vi "LV3Climb.vi"(7 "Deactivate?":bool, 8 "error in (no error)":errorcluster, 9 "Activate?":bool, 10 "Reclimb?":bool, 11 "Elevator Concrete in":refnum<class "Elevator Concrete.lvclass">) -> (0 "error out":errorcluster, 1 "activate wrist lock":bool, 3 "Elevator Concrete out":refnum<class "Elevator Concrete.lvclass">)   [LabVIEW 2018, in "Elevator.lvlib" / "Elevator Concrete.lvclass"]
uses:
  Elevator Concrete.lvclass
  C:/Users/Public/Documents/2019DeepSpace/Classes/Elevator/Elevator.lvclass
  Elevator States Climb.ctl
  Elevator.lvclass/Elevator.ctl
  <vilib>/Rock Robotics/WPI/ThirdParty/Phoenix-LabVIEW/Motor Controller/Controls/CTRE_Phoenix_MotorControl_ControlMode.ctl
  Elevator Concrete.lvclass/Elevator Concrete.ctl
  Public Methods/Read Arm Position Values.vi
  <vilib>/Rock Robotics/WPI/ThirdParty/Phoenix-LabVIEW/Motor Controller/Get/CTRE_Phoenix_MotorController_GetQuadratureData.vi
  <vilib>/Rock Robotics/Network Tables/NT Write String.vi
  Elevator.lvclass
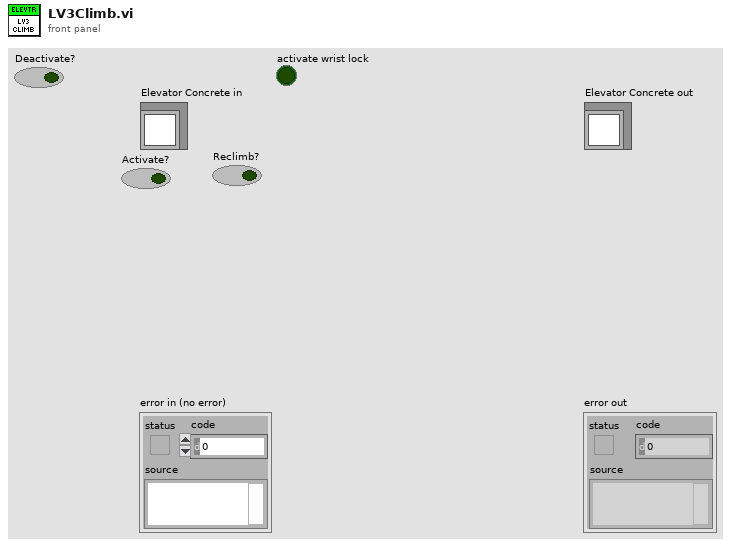
[diagram p1: front panel]
types:
  T1 = typedef "Elevator.lvlib/Elevator.lvclass/Elevator States Climb.ctl" = enum16{"Pre-Lift", "Deploy", "Activate Suction", "Climb", "Climbed", "Unclimb", ""}
  T2 = typedef "Elevator.lvlib/Elevator.lvclass/Elevator Constants.ctl" = cluster{"Arm Motion Magic Max Velocity":u32, "Arm Motion Magic Max Acceleration":u32, "Wrist Motion Magic Max Velocity":u32, "Wrist Motion Magic Max Acceleration":u32, "Arm Gear Ratio":dbl, "Wrist Gear Ratio":dbl, "Arm Encoder ABS Value":i32, "Wrist Encoder ABS Value":i32}
  T3 = typedef "Elevator.lvlib/Elevator.lvclass/Arm Position Values.ctl" = cluster{"C0 Arm":dbl, "C1 Arm":dbl, "C2 Arm":dbl, "H1 Arm":dbl, "H2 Arm":dbl, "C0 Wrist":dbl, "C1 Wrist ":dbl, "C2 Wrist":dbl, "H1 Wrist":dbl, "H2 Wrist":dbl, "Deploy Arm":dbl, "Deploy Wrist":dbl, "Climb Arm":dbl, "Climb Wrist":dbl, "Stowed Arm":dbl, "Stowed Wrist":dbl}
  T4 = typedef "CTRE_Phoenix_MotorControl_ControlMode.ctl" = u16
  T5 = typedef "WPI_MotorControlDeviceRef.ctl" = cluster{"DeviceStatus":errorcluster, "Type":T6, "PWM":cluster{"PWM Channel":T7, "DeadBand":T8}, "CAN":cluster{"Device Number":u8, "SetOutput VI Ref":variant, "GetOutput VI Ref":variant, "Enable VI Ref":variant, "Disable VI Ref":variant, "Data":variant}, "Invert":bool, "DIO PWM":cluster{"PWM \"Enable\" Channel":T7, "DIOChannel":T9, "PWM Rate":dbl}}
  T6 = typedef "WPI_MotorControlType.ctl" = enum16{"PWM", "CAN", "DIO PWM"}
  T7 = typedef "FPGA_DIOPWMChannel.ctl" = enum8{"PWM 0", "PWM 1", "PWM 2", "PWM 3", "PWM 4", "PWM 5", "PWM 6", "PWM 7", "PWM 8", "PWM 9", "PWM MXP 0", "PWM MXP 1", "PWM MXP 2", "PWM MXP 3", "PWM MXP 4", "PWM MXP 5", "PWM MXP 6", "PWM MXP 7", "PWM MXP 8", "PWM MXP 9", "Invalid"}
  T8 = typedef "WPI_PWMDeadband.ctl" = cluster{"Name":string, "maxPositivePwm":i32, "minPositivePwm":i32, "centerPwm":i32, "maxNegativePwm":i32, "minNegativePwm":i32, "angularRange":u16}
  T9 = typedef "FPGA_DIOChannel.ctl" = enum8{"DIO 0", "DIO 1", "DIO 2", "DIO 3", "DIO 4", "DIO 5", "DIO 6", "DIO 7", "DIO 8", "DIO 9", "DIO MXP 0", "DIO MXP 1", "DIO MXP 2", "DIO MXP 3", "DIO MXP 4", "DIO MXP 5", "DIO MXP 6", "DIO MXP 7", "DIO MXP 8", "DIO MXP 9", "DIO MXP 10", "DIO MXP 11", "DIO MXP 12", "DIO MXP 13", "DIO MXP 14", "DIO MXP 15", "SPI Port CS1", "SPI Port CS2", "SPI Port CS3", "SPI Port MISO", "SPI Port MOSI", "Invalid"}
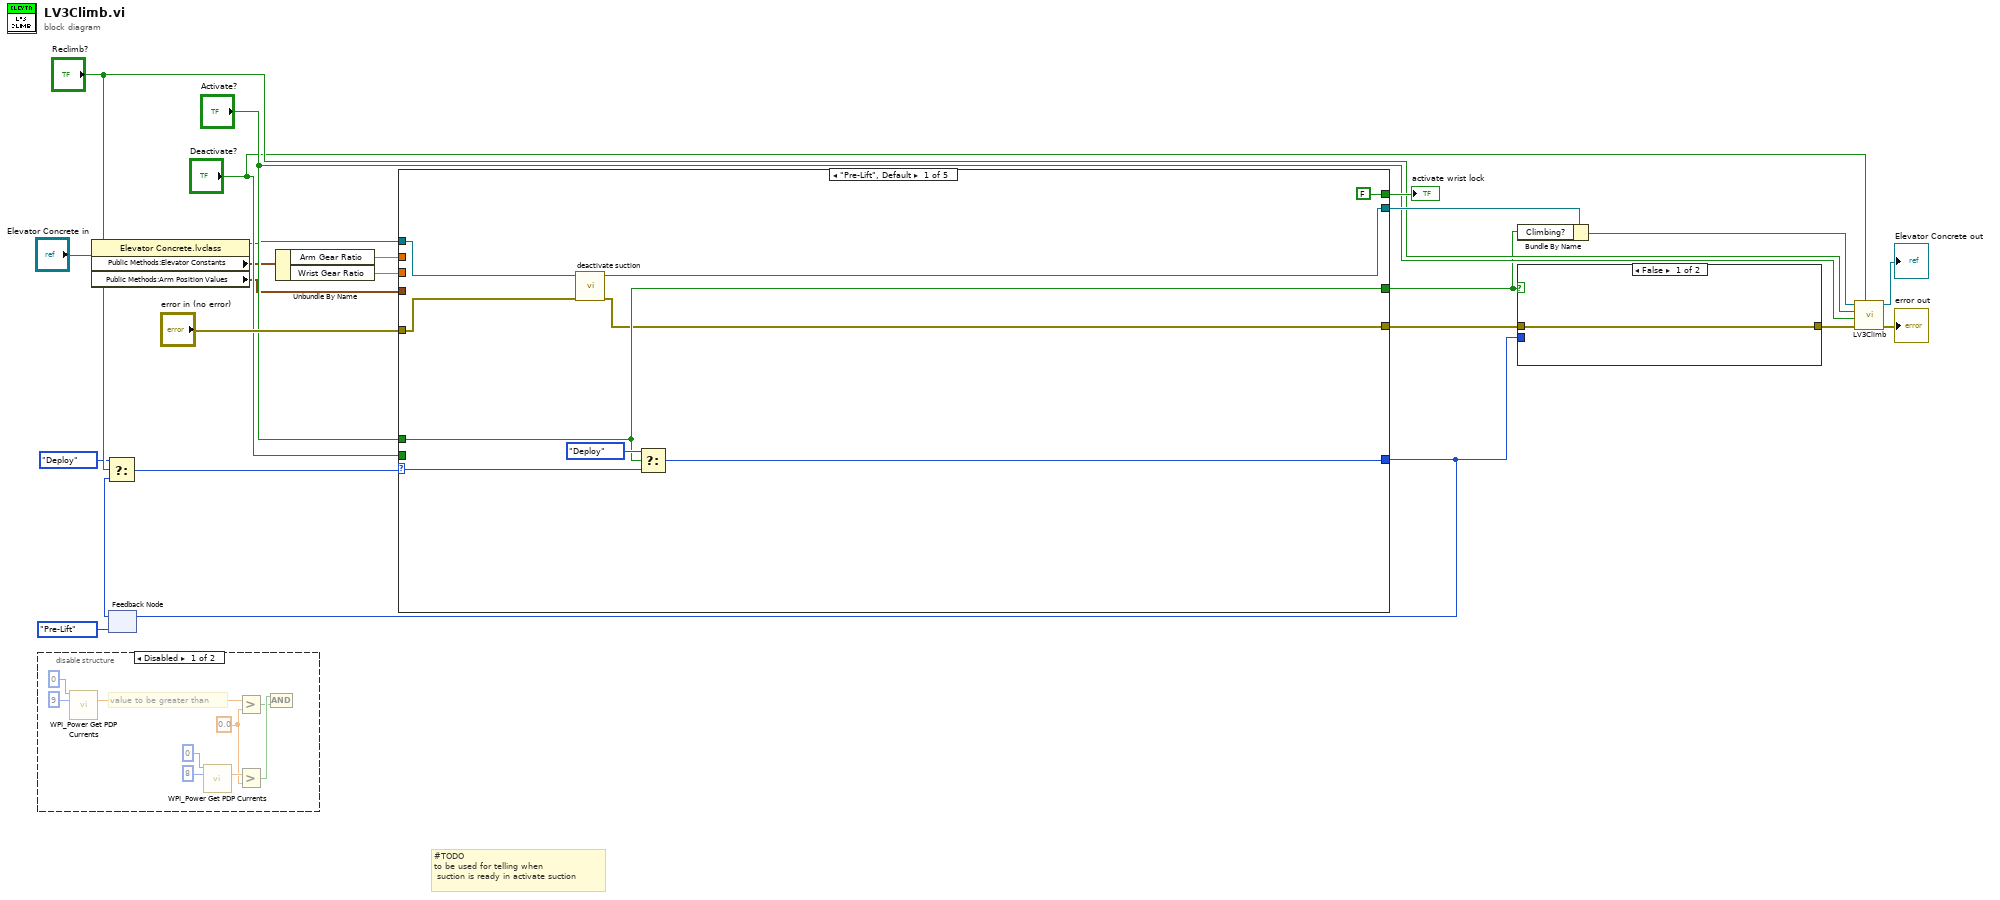
[diagram p0: block diagram]
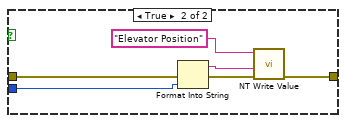
[diagram p2: hidden frame]
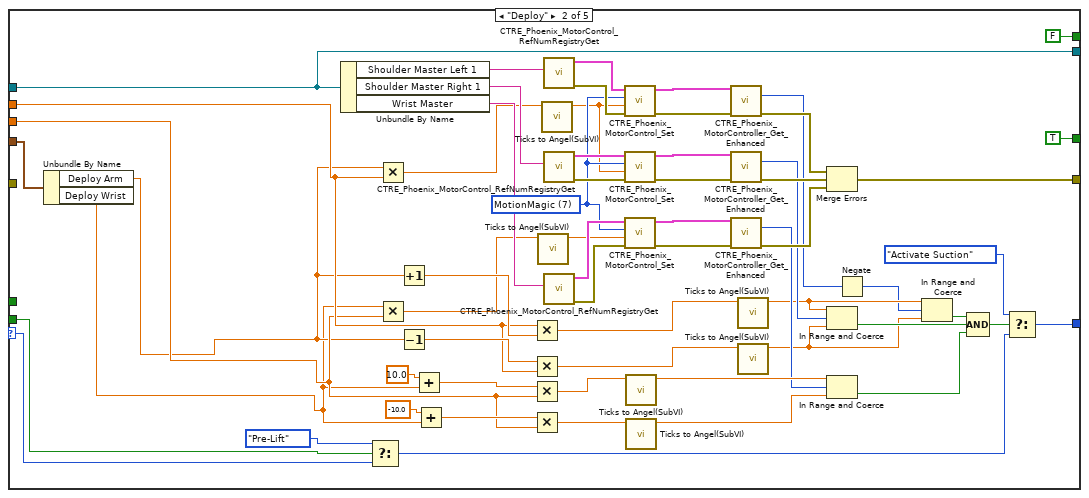
[diagram p4: hidden frame]
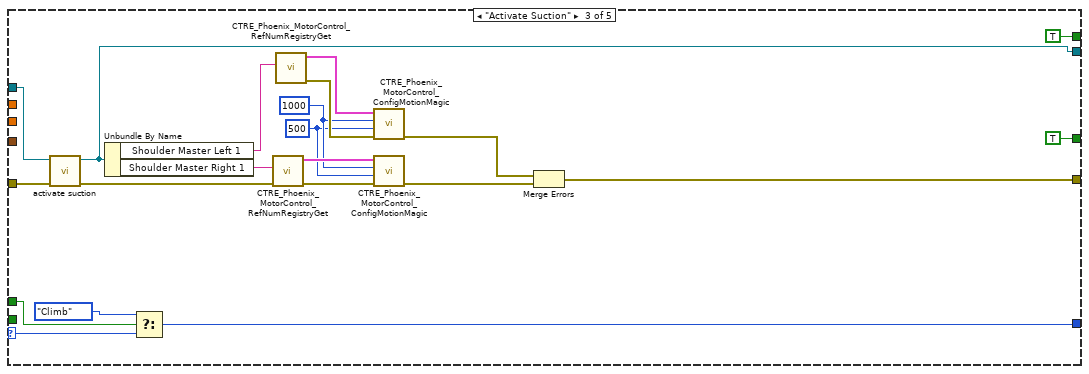
[diagram p5: hidden frame]
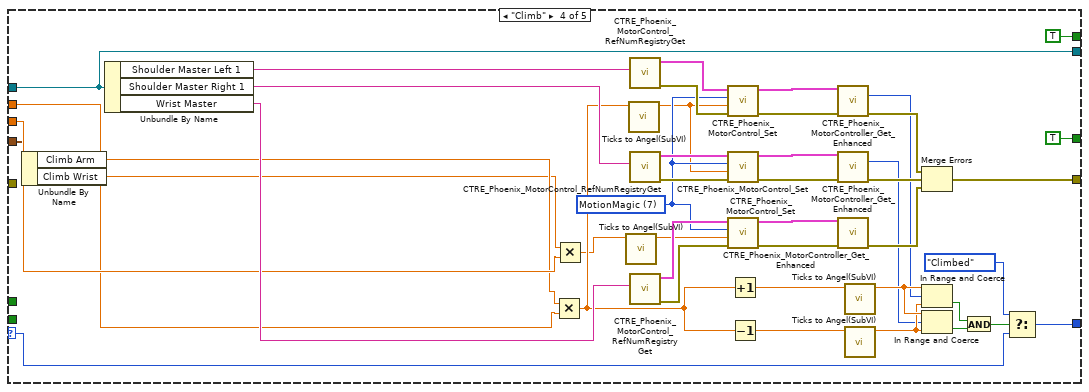
[diagram p6: hidden frame]
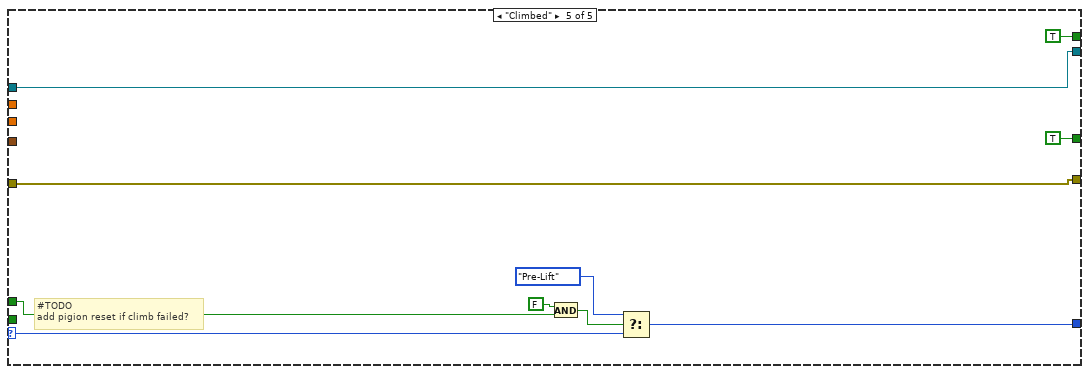
[diagram p7: hidden frame]
diagram:
  # "#TODO\nto be used for telling when\n suction is ready in activate suction"
  n1 = disable-structure shown="Disabled" {
    frame Disabled {
      w26 = 0.0
      # "value to be greater than"
      n2 = call <vilib>:"WPI_Power Get PDP Currents.vi"("Power Distribution Panel (0)"=u8 0, "PDP Channel"=9) -> ("current (A)"=w28:dbl)  [unwired: 11 in, 2 out]
      n3 = call <vilib>:"WPI_Power Get PDP Currents.vi"("Power Distribution Panel (0)"=u8 0, "PDP Channel"=8) -> ("current (A)"=w27:dbl)  [unwired: 11 in, 2 out]
      n4 = Greater?(x=w28, y=w26) -> (0:w24:bool)
      n5 = Greater?(x=w27, y=w26) -> (0:w25:bool)
      n6 = And(x=w25, y=w24) -> ()  [unwired: 1 out]
    }
    frame Enabled {
    }
  }
  n7 = property class="Elevator Concrete.lvclass"(reference="Elevator Concrete in") -> (reference out=w5:refnum<class "Elevator Concrete.lvclass">, "Public Methods:Elevator Constants"=w3:T2, "Public Methods:Arm Position Values"=w4:T3)  [unwired: 1 in, 1 out]
  n8 = feedback #1(Elevator_States_Climb."Pre-Lift") -> (w13:T1)
  n9 = Select(t=Elevator_States_Climb."Deploy", s="Reclimb?", f=w13) -> (s? t:f=w7:T1)
  n10 = Unbundle By Name(w3) -> ("Arm Gear Ratio"=w2:dbl, "Wrist Gear Ratio"=w1:dbl)
  n11 = case shown="\"Pre-Lift\", Default" w7 {
    selector: w7 -> [w40 w47 w119 w166 w169]
    tunnel: "Activate?" -> [w38 _ w116 _ w173]
    tunnel: w5 -> [w36 w101 w122 w161 w176]
    tunnel: [w35 w101 w115 w161 w176] -> w22
    tunnel: "error in (no error)" -> [w34 _ w121 _ w175]
    tunnel: [w33 w100 w107 w164 w175] -> w11
    tunnel: [w39 w99 w120 w165 w170] -> w9
    tunnel: [w38 TRUE TRUE TRUE TRUE] -> w8
    tunnel: [FALSE FALSE TRUE TRUE TRUE] -> w19
    tunnel: "Deactivate?" -> [_ w49 _ _ _]
    tunnel: w4 -> [_ w44 _ w125 _]
    tunnel: w2 -> [_ w46 _ w126 _]
    tunnel: w1 -> [_ w45 _ w127 _]
    frame "Pre-Lift", Default {
      n12 = call "deactivate suction.vi"("error in (no error)"=w34, "Elevator Concrete in"=w36) -> ("error out"=w33:errorcluster, "Elevator Concrete out"=w35:refnum<class "Elevator Concrete.lvclass">)  [unwired: 8 in]
      n13 = Select(t=Elevator_States_Climb."Deploy", s=w38, f=w40) -> (s? t:f=w39:T1)
    }
    frame "Deploy" {
      w77 = T4 7 items=["PercentOutput"=0, "Position"=1, "Velocity"=2, "Current"=3, "Follower"=5, "MotionProfile"=6, "MotionMagic"=7, "MotionProfileArc"=10, "Disabled"=15] ("Control Mode")
      n14 = Unbundle By Name(w44) -> ("Deploy Arm"=w43:dbl, "Deploy Wrist"=w42:dbl)
      n15 = Unbundle By Name(w101) -> ("Shoulder Master Left 1"=w76:string, "Shoulder Master Right 1"=w91:string, "Wrist Master"=w92:string)
      n16 = Select(t=Elevator_States_Climb."Pre-Lift", s=w49, f=w47) -> (s? t:f=w48:T1)
      n17 = Multiply(x=w43, y=w46) -> (x*y=w54:dbl)
      n18 = Multiply(x=w42, y=w45) -> (x*y=w59:dbl)
      n19 = Increment(x=w43) -> (x+1=w69:dbl)
      n20 = Decrement(x=w43) -> (x-1=w68:dbl)
      n21 = Add(x=10.0, y=w42) -> (x+y=w66:dbl)
      n22 = Add(x=-10.0, y=w42) -> (x+y=w65:dbl)
      n23 = Multiply(x=w46, y=w69) -> (x*y=w52:dbl)
      n24 = Multiply(x=w68, y=w46) -> (x*y=w53:dbl)
      n25 = Multiply(x=w66, y=w45) -> (x*y=w56:dbl)
      n26 = Multiply(x=w65, y=w45) -> (x*y=w55:dbl)
      n27 = call "Ticks to Angel(SubVI).vi"("Numeric in"=w59) -> ("Numeric out"=w82:dbl)  [unwired: 10 in]
      n28 = call "Ticks to Angel(SubVI).vi"("Numeric in"=w54) -> ("Numeric out"=w74:dbl)  [unwired: 10 in]
      n29 = call <vilib>:"CTRE_Phoenix_MotorControl_RefNumRegistryGet.vi"("refnum name"=w76) -> ("error out"=w79:errorcluster, "PhoenixMotorControlDevRef"=w81:T5)  [unwired: 9 in]
      n30 = call <vilib>:"CTRE_Phoenix_MotorControl_RefNumRegistryGet.vi"("refnum name"=w91) -> ("error out"=w96:errorcluster, "PhoenixMotorControlDevRef"=w95:T5)  [unwired: 9 in]
      n31 = call <vilib>:"CTRE_Phoenix_MotorControl_RefNumRegistryGet.vi"("refnum name"=w92) -> ("error out"=w93:errorcluster, "PhoenixMotorControlDevRef"=w94:T5)  [unwired: 9 in]
      n32 = call <vilib>:"CTRE_Phoenix_MotorControl_Set.vi"("error in (no error)"=w79, "Output"=w74, "Control Mode"=w77, "PhoenixMotorControlDevRef"=w81) -> ("error out"=w78:errorcluster, "PhoenixMotorControlDevRef"=w80:T5)  [unwired: 6 in]
      n33 = call <vilib>:"CTRE_Phoenix_MotorControl_Set.vi"("error in (no error)"=w96, "Output"=w74, "Control Mode"=w77, "PhoenixMotorControlDevRef"=w95) -> ("error out"=w86:errorcluster, "PhoenixMotorControlDevRef"=w87:T5)  [unwired: 6 in]
      n34 = call <vilib>:"CTRE_Phoenix_MotorControl_Set.vi"("error in (no error)"=w93, "Output"=w82, "Control Mode"=w77, "PhoenixMotorControlDevRef"=w94) -> ("error out"=w88:errorcluster, "PhoenixMotorControlDevRef"=w89:T5)  [unwired: 6 in]
      n35 = call "Ticks to Angel(SubVI).vi"("Numeric in"=w56) -> ("Numeric out"=w63:dbl)  [unwired: 10 in]
      n36 = call "Ticks to Angel(SubVI).vi"("Numeric in"=w55) -> ("Numeric out"=w64:dbl)  [unwired: 10 in]
      n37 = call-poly <vilib>:"CTRE_Phoenix_MotorController_Get_Enhanced.vi"("PhoenixMotorControlDevRef"=w80, "error in"=w78) -> ("Quadrature Position"=w70:i32, "error out"=w75:errorcluster)  [unwired: 10 in, 2 out]
      n38 = call-poly <vilib>:"CTRE_Phoenix_MotorController_Get_Enhanced.vi"("PhoenixMotorControlDevRef"=w87, "error in"=w86) -> ("Quadrature Position"=w67:i32, "error out"=w84:errorcluster)  [unwired: 10 in, 2 out]
      n39 = call-poly <vilib>:"CTRE_Phoenix_MotorController_Get_Enhanced.vi"("PhoenixMotorControlDevRef"=w89, "error in"=w88) -> ("Quadrature Position"=w62:i32, "error out"=w83:errorcluster)  [unwired: 10 in, 2 out]
      n40 = call "Ticks to Angel(SubVI).vi"("Numeric in"=w52) -> ("Numeric out"=w61:dbl)  [unwired: 10 in]
      n41 = call "Ticks to Angel(SubVI).vi"("Numeric in"=w53) -> ("Numeric out"=w60:dbl)  [unwired: 10 in]
      n42 = Merge Errors(w75, w84, w83) -> (w100:errorcluster)
      n43 = In Range and Coerce(upper limit=w61, x=w67, lower limit=w60) -> (In Range?=w72:bool)  [unwired: 1 out]
      n44 = In Range and Coerce(upper limit=w63, x=w62, lower limit=w64) -> (In Range?=w73:bool)  [unwired: 1 out]
      n45 = Negate(x=w70) -> (-x=w51:i32)
      n46 = In Range and Coerce(upper limit=w61, x=w51, lower limit=w60) -> (In Range?=w71:bool)  [unwired: 1 out]
      n47 = Compound Arithmetic op=AND(w71, w72, w73) -> (w85:bool)
      n48 = Select(t=Elevator_States_Climb."Activate Suction", s=w85, f=w48) -> (s? t:f=w99:T1)
    }
    frame "Activate Suction" {
      w104 = 1000 ("Cruise Velocity")
      w103 = 500 ("Acceleration")
      n49 = call "activate suction.vi"("error in (no error)"=w121, "Elevator Concrete in"=w122) -> ("error out"=w108:errorcluster, "Elevator Concrete out"=w115:refnum<class "Elevator Concrete.lvclass">)  [unwired: 8 in]
      n50 = Unbundle By Name(w115) -> ("Shoulder Master Left 1"=w113:string, "Shoulder Master Right 1"=w114:string)
      n51 = Select(t=Elevator_States_Climb."Climb", s=w116, f=w119) -> (s? t:f=w120:T1)
      n52 = call <vilib>:"CTRE_Phoenix_MotorControl_RefNumRegistryGet.vi"("error in (no error)"=w108, "refnum name"=w114) -> ("error out"=w112:errorcluster, "PhoenixMotorControlDevRef"=w111:T5)  [unwired: 8 in]
      n53 = call <vilib>:"CTRE_Phoenix_MotorControl_RefNumRegistryGet.vi"("refnum name"=w113) -> ("error out"=w110:errorcluster, "PhoenixMotorControlDevRef"=w109:T5)  [unwired: 9 in]
      n54 = call <vilib>:"CTRE_Phoenix_MotorControl_ConfigMotionMagic.vi"("error in (no error)"=w110, "Acceleration"=w103, "Cruise Velocity"=w104, "PhoenixMotorControlDevRef"=w109) -> ("error out"=w106:errorcluster)  [unwired: 6 in, 1 out]
      n55 = call <vilib>:"CTRE_Phoenix_MotorControl_ConfigMotionMagic.vi"("error in (no error)"=w112, "Acceleration"=w103, "Cruise Velocity"=w104, "PhoenixMotorControlDevRef"=w111) -> ("error out"=w105:errorcluster)  [unwired: 6 in, 1 out]
      n56 = Merge Errors(w106, w105) -> (w107:errorcluster)
    }
    frame "Climb" {
      w143 = T4 7 items=["PercentOutput"=0, "Position"=1, "Velocity"=2, "Current"=3, "Follower"=5, "MotionProfile"=6, "MotionMagic"=7, "MotionProfileArc"=10, "Disabled"=15] ("Control Mode")
      n57 = Unbundle By Name(w125) -> ("Climb Arm"=w124:dbl, "Climb Wrist"=w123:dbl)
      n58 = Unbundle By Name(w161) -> ("Shoulder Master Left 1"=w142:string, "Shoulder Master Right 1"=w155:string, "Wrist Master"=w156:string)
      n59 = Multiply(x=w124, y=w126) -> (x*y=w129:dbl)
      n60 = Multiply(x=w123, y=w127) -> (x*y=w128:dbl)
      n61 = call "Ticks to Angel(SubVI).vi"("Numeric in"=w128) -> ("Numeric out"=w130:dbl)  [unwired: 10 in]
      n62 = call "Ticks to Angel(SubVI).vi"("Numeric in"=w129) -> ("Numeric out"=w131:dbl)  [unwired: 10 in]
      n63 = call <vilib>:"CTRE_Phoenix_MotorControl_RefNumRegistryGet.vi"("refnum name"=w142) -> ("error out"=w145:errorcluster, "PhoenixMotorControlDevRef"=w147:T5)  [unwired: 9 in]
      n64 = call <vilib>:"CTRE_Phoenix_MotorControl_RefNumRegistryGet.vi"("refnum name"=w155) -> ("error out"=w160:errorcluster, "PhoenixMotorControlDevRef"=w159:T5)  [unwired: 9 in]
      n65 = call <vilib>:"CTRE_Phoenix_MotorControl_RefNumRegistryGet.vi"("refnum name"=w156) -> ("error out"=w157:errorcluster, "PhoenixMotorControlDevRef"=w158:T5)  [unwired: 9 in]
      n66 = call <vilib>:"CTRE_Phoenix_MotorControl_Set.vi"("error in (no error)"=w145, "Output"=w131, "Control Mode"=w143, "PhoenixMotorControlDevRef"=w147) -> ("error out"=w144:errorcluster, "PhoenixMotorControlDevRef"=w146:T5)  [unwired: 6 in]
      n67 = call <vilib>:"CTRE_Phoenix_MotorControl_Set.vi"("error in (no error)"=w160, "Output"=w131, "Control Mode"=w143, "PhoenixMotorControlDevRef"=w159) -> ("error out"=w151:errorcluster, "PhoenixMotorControlDevRef"=w152:T5)  [unwired: 6 in]
      n68 = call <vilib>:"CTRE_Phoenix_MotorControl_Set.vi"("error in (no error)"=w157, "Output"=w130, "Control Mode"=w143, "PhoenixMotorControlDevRef"=w158) -> ("error out"=w153:errorcluster, "PhoenixMotorControlDevRef"=w154:T5)  [unwired: 6 in]
      n69 = Increment(x=w129) -> (x+1=w139:dbl)
      n70 = Decrement(x=w129) -> (x-1=w138:dbl)
      n71 = call-poly <vilib>:"CTRE_Phoenix_MotorController_Get_Enhanced.vi"("PhoenixMotorControlDevRef"=w146, "error in"=w144) -> ("Quadrature Position"=w134:i32, "error out"=w141:errorcluster)  [unwired: 10 in, 2 out]
      n72 = call-poly <vilib>:"CTRE_Phoenix_MotorController_Get_Enhanced.vi"("PhoenixMotorControlDevRef"=w152, "error in"=w151) -> ("Quadrature Position"=w135:i32, "error out"=w149:errorcluster)  [unwired: 10 in, 2 out]
      n73 = call-poly <vilib>:"CTRE_Phoenix_MotorController_Get_Enhanced.vi"("PhoenixMotorControlDevRef"=w154, "error in"=w153) -> ("error out"=w148:errorcluster)  [unwired: 10 in, 3 out]
      n74 = call "Ticks to Angel(SubVI).vi"("Numeric in"=w139) -> ("Numeric out"=w137:dbl)  [unwired: 10 in]
      n75 = call "Ticks to Angel(SubVI).vi"("Numeric in"=w138) -> ("Numeric out"=w136:dbl)  [unwired: 10 in]
      n76 = Merge Errors(w141, w149, w148) -> (w164:errorcluster)
      n77 = In Range and Coerce(upper limit=w137, x=w134, lower limit=w136) -> (In Range?=w132:bool)  [unwired: 1 out]
      n78 = In Range and Coerce(upper limit=w137, x=w135, lower limit=w136) -> (In Range?=w133:bool)  [unwired: 1 out]
      n79 = And(x=w132, y=w133) -> (x .and. y?=w150:bool)
      n80 = Select(t=Elevator_States_Climb."Climbed", s=w150, f=w166) -> (s? t:f=w165:T1)
    }
    frame "Climbed" {
      # "#TODO\nadd pigion reset if climb failed?"
      n81 = And(x=FALSE, y=w173) -> (x .and. y?=w174:bool)
      n82 = Select(t=Elevator_States_Climb."Pre-Lift", s=w174, f=w169) -> (s? t:f=w170:T1)
    }
  }
  "activate wrist lock" <- w19
  n83 = feedback-in #1(w9) -> ()
  n84 = Bundle By Name(cluster=w22, "Climbing?"=w8) -> (w18:refnum<class "Elevator Concrete.lvclass">)
  n85 = case shown="False" w8 {
    tunnel: [w177 w180] -> w10
    tunnel: w11 -> [w177 w179]
    tunnel: w9 -> [_ w178]
    frame False {
    }
    frame True {
      n86 = Format Into String(error in=w179, w178) -> (resulting string=w182:string, error out=w181:errorcluster)  [unwired: 2 in]
      n87 = call-poly <vilib>:"NT Write Value.vi"("error in"=w181, "String"=w182, "Name"="Elevator Position") -> ("error out"=w180:errorcluster)  [unwired: 8 in]
    }
  }
  n88 = call-parent "LV3Climb.vi"("Deactivate?"="Deactivate?", "error in (no error)"=w10, "Activate?"="Activate?", "Redeploy?"="Reclimb?", "Elevator in"=w18) -> ("error out"=→"error out":errorcluster, "Elevator out"=→"Elevator Concrete out":refnum<class "Elevator Concrete.lvclass">)  [unwired: 4 in, 1 out]
